vi "Send Command.vi"(8 "error in (no error)":errorcluster, 9 "Expected Response":string, 10 "Command":string, 11 "Serial Device":refnum<class "Serial Device.lvclass">) -> (0 "error out":errorcluster, 2 "read buffer":string, 3 "Serial Device Out":refnum<class "Serial Device.lvclass">)   [LabVIEW 2017, in "Serial Device.lvclass"]
uses:
  Serial Device.lvclass
  Serial Device.lvclass/Serial Device.ctl
  Get Serial Port.vi
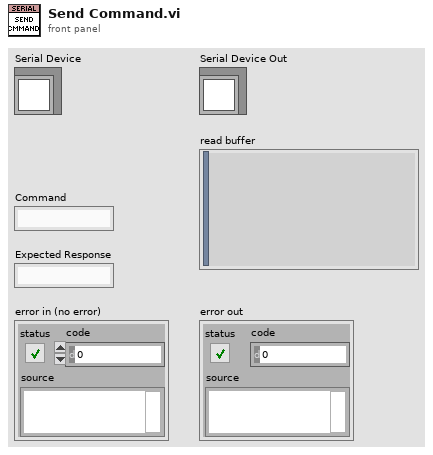
[diagram p1: front panel]
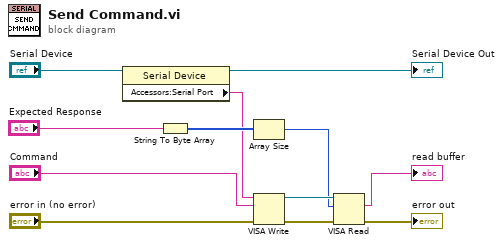
[diagram p0: block diagram]
diagram:
  n1 = property class="Serial Device"(reference="Serial Device") -> (reference out=→"Serial Device Out":refnum<class "Serial Device.lvclass">, "Accessors:Serial Port"=w2:string)  [unwired: 1 in, 1 out]
  n2 = String To Byte Array(string="Expected Response") -> (unsigned byte array=w8:u8[])
  n3 = Array Size(array=w8) -> (size(s)=w9:i32)
  n4 = VISA Write(VISA resource name=w2, write buffer="Command", error in (no error)="error in (no error)") -> (VISA resource name out=w12:refnum<visa-resource-name>, error out=w6:errorcluster)  [unwired: 1 out]
  n5 = VISA Read(VISA resource name=w12, byte count=w9, error in (no error)=w6) -> (read buffer=→"read buffer":string, error out=→"error out":errorcluster)  [unwired: 2 out]
